vi "Fibonacci_series_modified.vi"() -> ()   [LabVIEW 2019]
panel:
  in  "stop":bool
  out "Fibonocci Series":u64[](array[numeric])
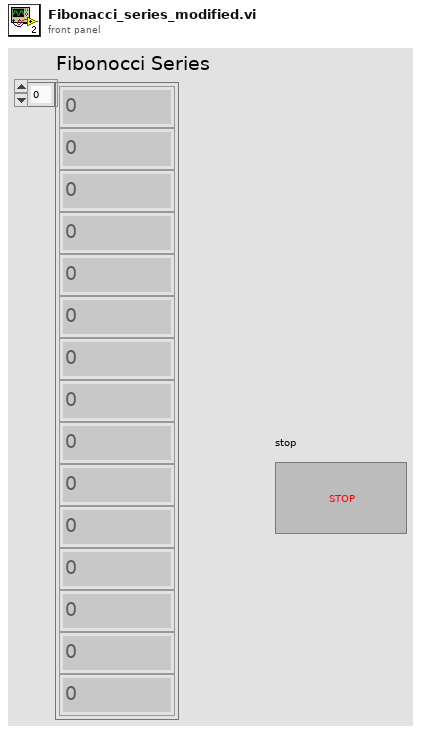
[diagram p1: front panel]
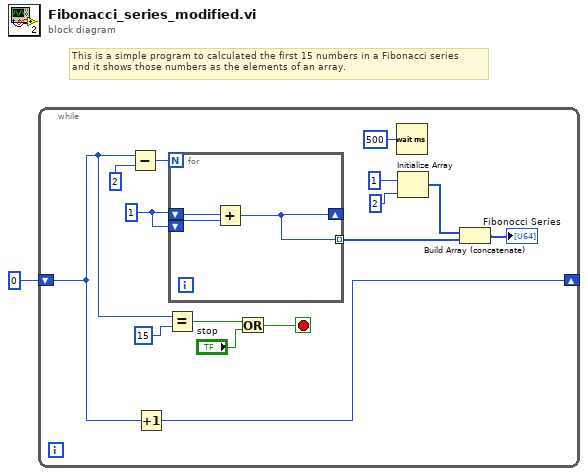
[diagram p0: block diagram]
diagram:
  # "This is a simple program to calculated the first 15 numbers in a Fibonacci series\nand it shows those numbers as the elements of an array."
  n1 = while {
    shift-right: [w7] -> _
    shift-left: 0 -> [w2]
    stop <- w3 stop-if-true
    w16 = u64 1
    n2 = Subtract(x=w2, y=2 ("dimension size")) -> (x-y=w13:i32)
    n3 = Increment(x=w2) -> (x+1=w7:i32)
    n4 = Equal?(x=w2, y=15) -> (x = y?=w5:bool)
    n5 = for {
      N: w13 -> [_]
      shift-right: [w19] -> _
      shift-left: w16 -> [w17]
      shift-left: w16 -> [w18]
      tunnel: [w19] -> w10 mode=indexing
      n6 = Add(x=w17, y=w18) -> (x+y=w19:u64)
    }
    n7 = Or(x=w5, y="stop") -> (x .or. y?=w3:bool)
    n8 = Wait (ms)(milliseconds to wait=u32 500) -> ()  [unwired: 1 out]
    n9 = Initialize Array(u64 1, 2 ("dimension size")) -> (w11:u64[])
    n10 = Build Array (concatenate)(w11, w10) -> (→"Fibonocci Series":u64[])
  }
